vi "MPExxx_set_curr.vi"(2 "error in (no error)":errorcluster, 3 "Set Current":dbl format="%.2f", 4 "VISA session":refnum<visa-resource-name>) -> (0 "error out":errorcluster, 1 "dup VISA session":refnum<visa-resource-name>)   [LabVIEW 2023]
doc: "These VI form sets the immediate current level of the power supply."
panel:
  # "MAGNA-POWER"
  # "Electronics"
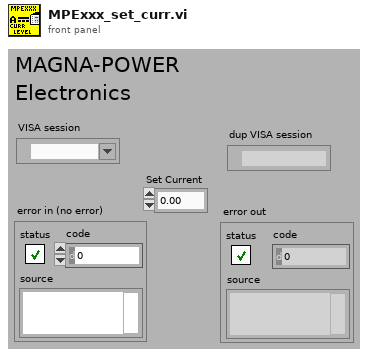
[diagram p1: front panel]
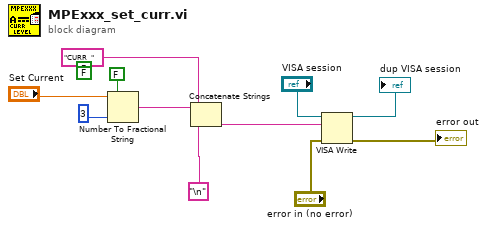
[diagram p0: block diagram]
diagram:
  (unwired) FALSE ("use system decimal point (T)")
  (unwired) FALSE ("use system decimal point (T)")
  n1 = Number To Fractional String(use system decimal point (T)=FALSE, number="Set Current", precision (6)=3) -> (F-format string=w6:string)  [unwired: 1 in]
  n2 = Concatenate Strings("CURR  ", w6, "\n") -> (w10:string)
  n3 = VISA Write(VISA resource name="VISA session", write buffer=w10, error in (no error)="error in (no error)") -> (VISA resource name out=→"dup VISA session":refnum<visa-resource-name>, error out=→"error out":errorcluster)  [unwired: 1 out]
